vi "SPD.Detector Connection Test.vi"(8 "Error In":errorcluster, 11 "SPD.Stand Ctrl in":T1 {"spdDeviceSession"."hidSPD.Controller"."HV_bias" format="%#_6p, V"; "spdDeviceSession"."hidSPD.Controller"."TSet" format="%#_6p, DegC"}) -> (0 "Error Out":errorcluster, 1 "HW ok":bool, 2 "HW report":string, 3 "SPD.Stand Ctrl out":T1 {"spdDeviceSession"."hidSPD.Controller"."HV_bias" format="%#_6p, V"; "spdDeviceSession"."hidSPD.Controller"."TSet" format="%#_6p, DegC"})   [LabVIEW 2018]
uses:
  typedefs/SPD.Stand Ctrl.ctl
  Instruments/SPD HID Interface/hidSPDLibForLabView/LibVIs/hidSPD Controls/hidSPD Device Session.ctl
  Instruments/SPD HID Interface/hidSPDLibForLabView/LibVIs/hidSPD Controls/hidSPD Controller.ctl
  Instruments/KC705 DevBoard/typedefs/DevB.Session.ctl
  Instruments/KeySight 53230A/typedefs/FreqC.Session.ctl
  Instruments/KeySight 8164B/KeySight 8164B LAN InstrLib/typedefs/KeySight 8164B control.ctl
  Instruments/LeCroy SDA830/typedefs/LeCroy.Session.ctl
  typedefs/SPD.Events.ctl
  <vilib>/Utility/config.llb/Config Data RefNum.ctl
  typedefs/SPD.Meas Result.ctl
  Instruments/SPD HID Interface/hidSPDLibForLabView/LibVIs/hidSPD Controls/hidSPD Controller Setup Report.ctl
  Instruments/SPD HID Interface/hidSPDLibForLabView/LibVIs/hidSPD Read Report/hidSPD Read SPD Name.vi
  Instruments/SPD HID Interface/hidSPDLibForLabView/LibVIs/hidSPD Write Report/hidSPD Setup Controller.vi
  Instruments/SPD HID Interface/hidSPDLibForLabView/hidSPDLibForLabView.lvlib
  Instruments/KeySight 8164B/KeySight 8164B LAN InstrLib.lvlib
  <vilib>/Utility/config.llb/NI_LVConfig.lvlib
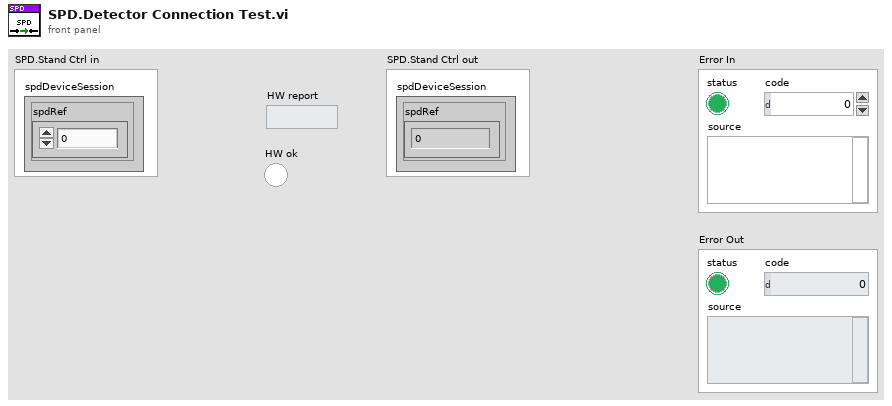
[diagram p1: front panel]
types:
  T1 = typedef "SPD.Stand Ctrl.ctl" = cluster{"spdDeviceSession":T2, "DevBSession":T4, "FreqCSession":T5, "8164BSession":T6, "LeCroySession":T7, "Events":T8, "configFile":T9, "SPD.Result":T10}
  T2 = typedef "hidSPDLibForLabView.lvlib/hidSPD Device Session.ctl" = cluster{"spdRef":u64, "connected":bool, "spdName":string, "hidSPD.Controller":T3}
  T3 = typedef "hidSPDLibForLabView.lvlib/hidSPD Controller.ctl" = cluster{"TSet":sgl, "HV_bias":sgl, "DDS_stb_code":u16}
  T4 = typedef "DevB.Session.ctl" = cluster{"DevBRef":refnum<visa-resource-name>, "connected":bool}
  T5 = typedef "FreqC.Session.ctl" = cluster{"FreqCRef":refnum<visa-resource-name>, "timeout":dbl, "Gate":dbl, "connected":bool}
  T6 = typedef "KeySight 8164B LAN InstrLib.lvlib/KeySight 8164B control.ctl" = cluster{"Connection ID":refnum<k5>, "Connected":bool, "Info":string, "Slots Info":string[]}
  T7 = typedef "LeCroy.Session.ctl" = cluster{"LeCroySession":refnum<visa-resource-name>, "connected":bool}
  T8 = typedef "SPD.Events.ctl" = cluster{"DCRTest":refnum<user-event>, "Stop":refnum<user-event>}
  T9 = typedef "NI_LVConfig.lvlib/Config Data RefNum.ctl" = refnum<k1>
  T10 = typedef "SPD.Meas Result.ctl" = cluster{"HV_Bias":dbl[][][], "Stb_code":dbl[], "Temprature":dbl[], "Data":dbl[][][][]}
  T11 = typedef "hidSPDLibForLabView.lvlib/hidSPD Controller Setup Report.ctl" = cluster{"TSet":sgl, "HV_bias":sgl, "DDS_stb_code":u16, "SPD_reset":u16, "MCU_reset":u16}
  T12 = typedef "hidSPDLibForLabView.lvlib/hidSPD HidDevInfo.ctl" = cluster{"name":string, "path":string}
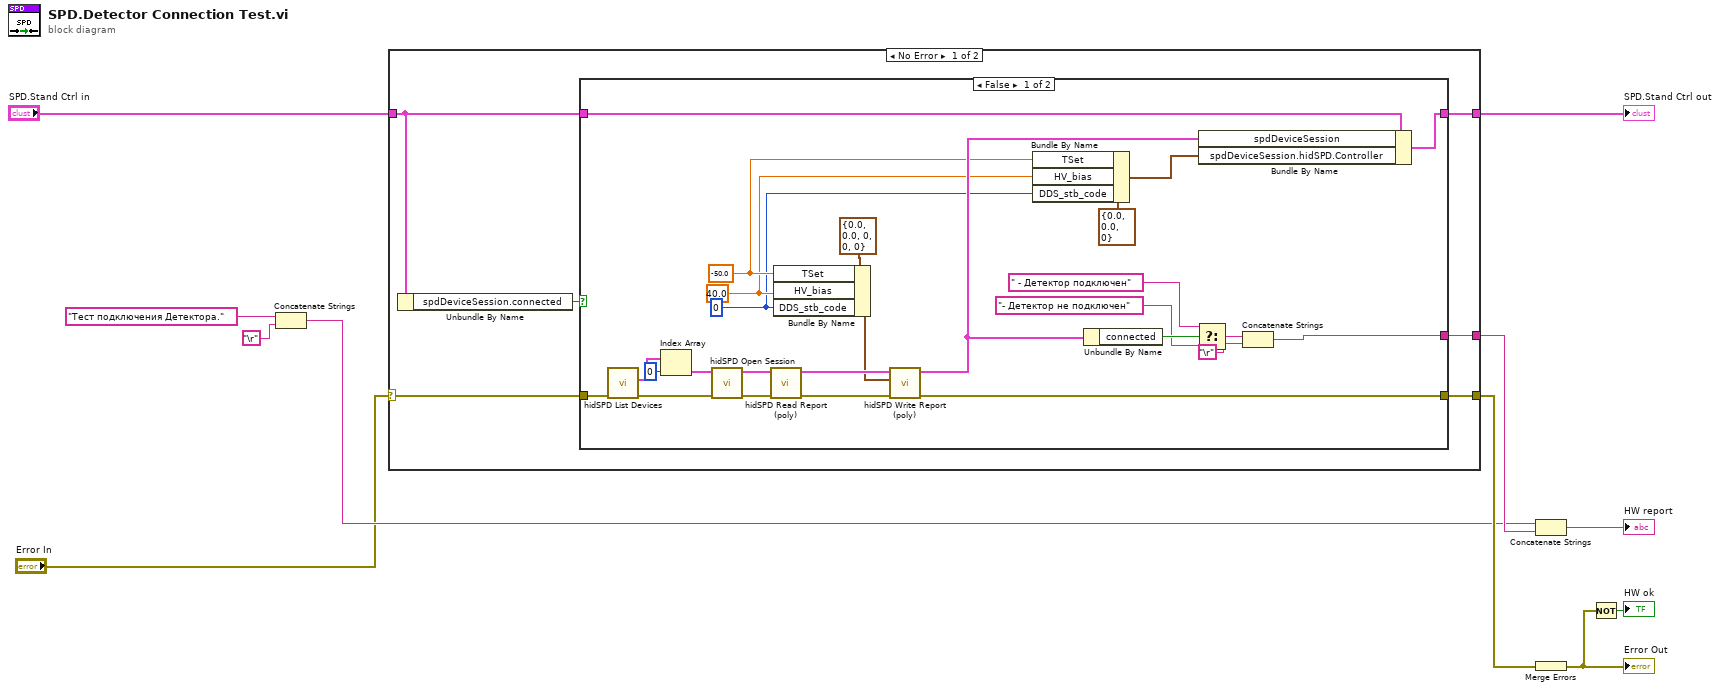
[diagram p0: block diagram]
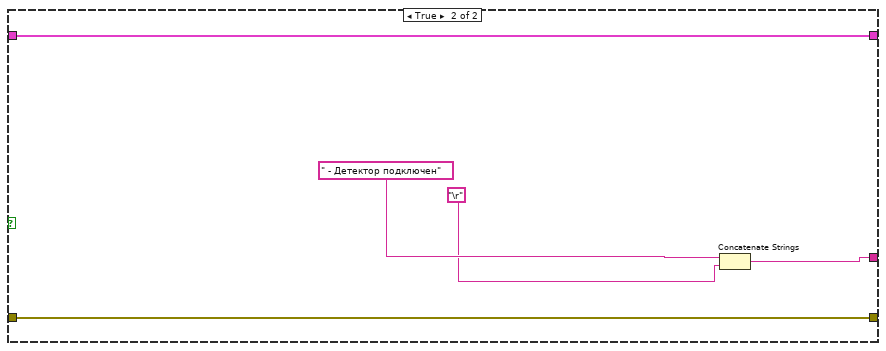
[diagram p2: hidden frame]
diagram:
  n1 = Concatenate Strings("Тест подключения Детектора.", "\r") -> (w4:string)
  n2 = case shown="No Error" "Error In" {
    selector: "Error In" -> [w15 w49]
    tunnel: "SPD.Stand Ctrl in" -> [w13 w50]
    tunnel: [w14 w49] -> w9
    tunnel: [w17 w50] -> w1
    tunnel: [w16 _] -> w11
    frame No Error {
      n3 = Unbundle By Name(w13) -> ("spdDeviceSession.connected"=w12:bool)
      n4 = case shown="False" w12 {
        tunnel: w13 -> [w43 w48]
        tunnel: [w39 w48] -> w17
        tunnel: [w37 w45] -> w16
        tunnel: w15 -> [w35 w47]
        tunnel: [w24 w47] -> w14
        frame False {
          w19 = u16 0 ("DDS_stb_code")
          w20 = sgl 40.0 ("HV_bias")
          w21 = sgl -50.0 ("TSet")
          n5 = call "hidSPD List Devices.vi"("error in (no error)"=w35) -> ("error out"=w31:errorcluster, "devices list"=w34:T12[])  [unwired: 9 in]
          n6 = Index Array(array=w34, index=0) -> (element=w32:T12)
          n7 = call "hidSPD Open Session.vi"("error in (no error)"=w31, "HidDevInfo"=w32) -> ("error out"=w29:errorcluster, "spdDevSession out"=w30:T2)  [unwired: 8 in]
          n8 = call-poly "hidSPD Read Report (poly).vi"("error in (no error)"=w29, "spdDevSession in"=w30) -> ("error out"=w25:errorcluster, "spdDevSession out"=w27:T2)  [unwired: 7 in, 1 out]
          n9 = Bundle By Name(cluster=T11 {"TSet"=0.0, "HV_bias"=0.0, "DDS_stb_code"=0, "SPD_reset"=0, "MCU_reset"=0} ("hidSPD Controller Setup report"), "TSet"=w21, "HV_bias"=w20, "DDS_stb_code"=w19) -> (w22:T11)
          n10 = call-poly "hidSPD Write Report (poly).vi"("error in (no error)"=w25, "hidSPD Controller Setup report"=w22, "spdDevSession in"=w27) -> ("error out"=w24:errorcluster, "spdDevSession out"=w26:T2)  [unwired: 7 in]
          n11 = Bundle By Name(cluster=T3 {"TSet"=0.0, "HV_bias"=0.0, "DDS_stb_code"=0} ("spdDeviceSession.hidSPD.Controller"), "TSet"=w21, "HV_bias"=w20, "DDS_stb_code"=w19) -> (w18:T3)
          n12 = Unbundle By Name(w26) -> ("connected"=w42:bool)
          n13 = Select(t=" - Детектор подключен", s=w42, f="- Детектор не подключен") -> (s? t:f=w38:string)
          n14 = Bundle By Name(cluster=w43, "spdDeviceSession"=w26, "spdDeviceSession.hidSPD.Controller"=w18) -> (w39:T1)
          n15 = Concatenate Strings(w38, "\r") -> (w37:string)
        }
        frame True {
          n16 = Concatenate Strings(" - Детектор подключен", "\r") -> (w45:string)
        }
      }
    }
    frame Error {
    }
  }
  "SPD.Stand Ctrl out" <- w1
  n17 = Concatenate Strings(w4, w11) -> (→"HW report":string)
  n18 = Merge Errors(w9) -> (w8:errorcluster)
  "Error Out" <- w8
  n19 = Not(x=w8) -> (.not. x?=→"HW ok":bool)
